vi "SetModeSweepTx.vi"(7 "Full-Sweep?":bool, 8 "error in (no error)":errorcluster, 10 "TxFrequencies":dbl[](array[numeric]) format="%.2f", 11 "Frequency Step":dbl format="%.2f") -> (0 "error out":errorcluster)   [LabVIEW 2011]
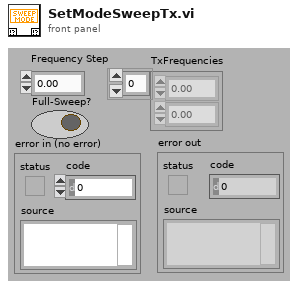
[diagram p1: front panel]
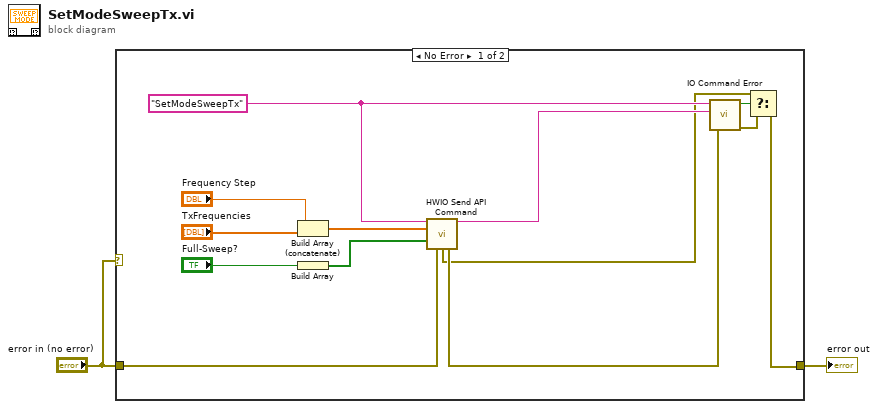
[diagram p0: block diagram]
diagram:
  n1 = case shown="No Error" "error in (no error)" {
    tunnel: "error in (no error)" -> [w15 w16]
    tunnel: [w9 w16] -> w2
    frame No Error {
      w13 = "SetModeSweepTx"
      n2 = Build Array (concatenate)("Frequency Step", "TxFrequencies") -> (w5:dbl[])
      n3 = Build Array("Full-Sweep?") -> (w3:bool[])
      n4 = call "HWIO Send API Command.vi"("Action"=w13, "Double"=w5, "Boolean"=w3, "error in (no error)"=w15) -> ("Action out"=w12:string, "HWError"=w8:errorcluster, "error out"=w14:errorcluster)  [unwired: 4 in, 5 out]
      n5 = call "IO Command Error.vi"("error in (no error)"=w14, "Command Returned (\"\")"=w12, "Command Sent (\"\")"=w13) -> ("error out"=w10:errorcluster, "HW ERR?"=w11:bool)  [unwired: 3 out]
      n6 = Select(t=w8, s=w11, f=w10) -> (s? t:f=w9:errorcluster)
    }
    frame Error {
    }
  }
  "error out" <- w2
